vi "Read new s4 acq config.vi"(8 "error in (no error)":errorcluster, 11 "SPARC4_Channel in":refnum<class "ECHARPE_Channel.lvclass">) -> (0 "error out":errorcluster, 1 "new acq config":cluster{"suffix":string, "#CYCLES":u32}, 2 "new s4 acq config":T1={"#SEQS"=1, "WAVEPLATE_POS"=0, "Waveplate positions"=[]}, 3 "SPARC4_Channel out":refnum<class "ECHARPE_Channel.lvclass">)   [LabVIEW 2018, in "ECHARPE_Channel.lvclass"]
uses:
  ECHARPE_Channel.lvclass
  ECHARPE_Channel.lvclass/ECHARPE_Channel.ctl
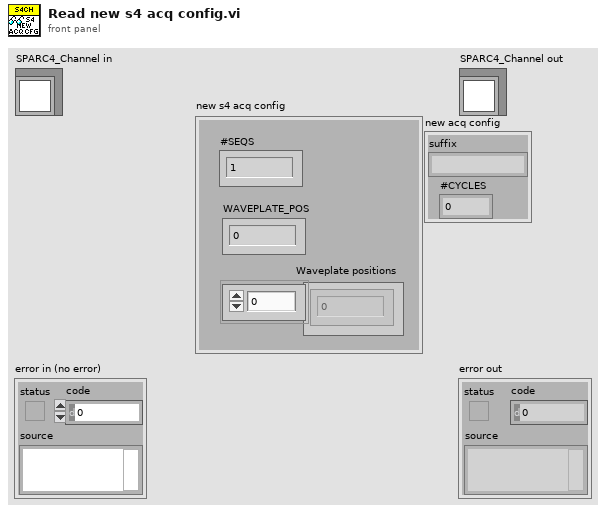
[diagram p1: front panel]
types:
  T1 = cluster{"#SEQS":u32, "WAVEPLATE_POS":i32, "Waveplate positions":u8[]}
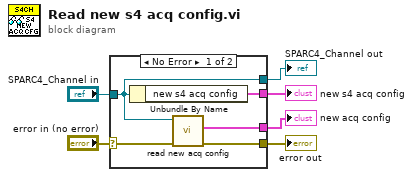
[diagram p0: block diagram]
diagram:
  n1 = case shown="No Error" "error in (no error)" {
    selector: "error in (no error)" -> [w10 w12]
    tunnel: [w8 w12] -> w5
    tunnel: [w9 w13] -> w3
    tunnel: "SPARC4_Channel in" -> [w9 w13]
    tunnel: [w11 _] -> w2
    tunnel: [w7 _] -> w1
    frame No Error {
      n2 = Unbundle By Name(w9) -> ("new s4 acq config"=w11:T1)
      n3 = call-dynamic "read new acq config.vi"("error in (no error)"=w10, "Channel in"=w9) -> ("error out"=w8:errorcluster, "new acq config"=w7:cluster{"suffix":string, "#CYCLES":u32})  [unwired: 7 in, 1 out]
    }
    frame Error {
    }
  }
  "error out" <- w5
  "SPARC4_Channel out" <- w3
  "new s4 acq config" <- w2
  "new acq config" <- w1
